vi "save vi front panel image.vi"(8 "error in (no error)":errorcluster, 10 "path to JPEG file":path, 11 "This VI":refnum<vi>) -> (0 "error out":errorcluster)   [LabVIEW 2013]
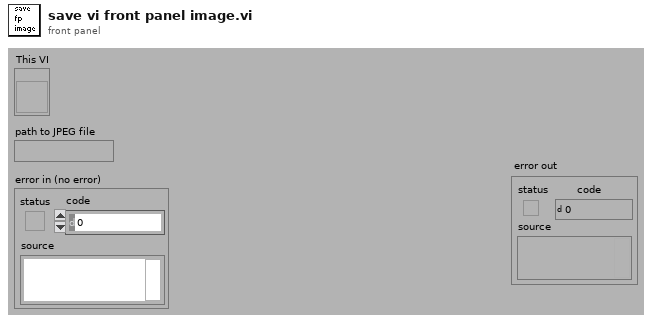
[diagram p1: front panel]
types:
  T1 = typedef "imagedata.ctl" = cluster{"image type":i32, "image depth":i32, "image":u8[], "mask":u8[], "colors":u32[], "Rectangle":cluster{"left":i16, "top":i16, "right":i16, "bottom":i16}}
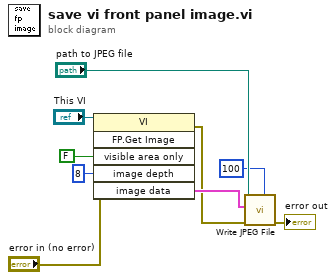
[diagram p0: block diagram]
diagram:
  n1 = invoke class="VI" method="FP.Get Image"(reference="This VI", error in="error in (no error)", "visible area only"=FALSE ("Visible Area Only"), "image depth"=8 ("Image Depth")) -> (error out=w5:errorcluster, "image data"=w6:T1)  [unwired: 2 in, 4 out]
  n2 = call <vilib>:"Write JPEG File.vi"("quality (80)"=100, "error in (no error)"=w5, "image data"=w6, "path to JPEG file"="path to JPEG file") -> ("error out"=→"error out":errorcluster)  [unwired: 6 in, 1 out]
